vi "TSM SSC Digital Apply TDR Offsets Per-Site Per-Pin.vi"(0 "Digital TSM In":T1, 5 "Per-Site Per-Pin TDR Values":dbl[][](array[numeric]) format="%#_6p", 11 "error in":errorcluster) -> (4 "Digital TSM Out":T1, 15 "error out":errorcluster)   [LabVIEW 2020]
doc: "Applies the correction for propagation delay offsets to a digital pattern instrument. Use this VI to apply TDR offsets that are stored from a past measurement or are measured by means other than the niDigital TDR VI. Also use this VI to apply correction for offsets if the <B>apply offsets</B> input of the niDigital TDR VI was set to False at the time of measurement."
uses:
  TSM/TSM SSC Digital.ctl
  <vilib>/NI_TestStand_SemiconductorModule/NI_TestStand_Semiconductor_Module.lvlibp/PinMap/Digital Pattern/PinQueryContext/DigitalPatternPinQueryContext.lvclass
  SSC Digital/SSC Digital.ctl
  1a9f9ff5-721a-42b6-b454-8659b893b2e8.vi
  Shared SubVIs/Channel List to Pins.vi
  Shared SubVIs/Trim Whitespace [Inlined].vi
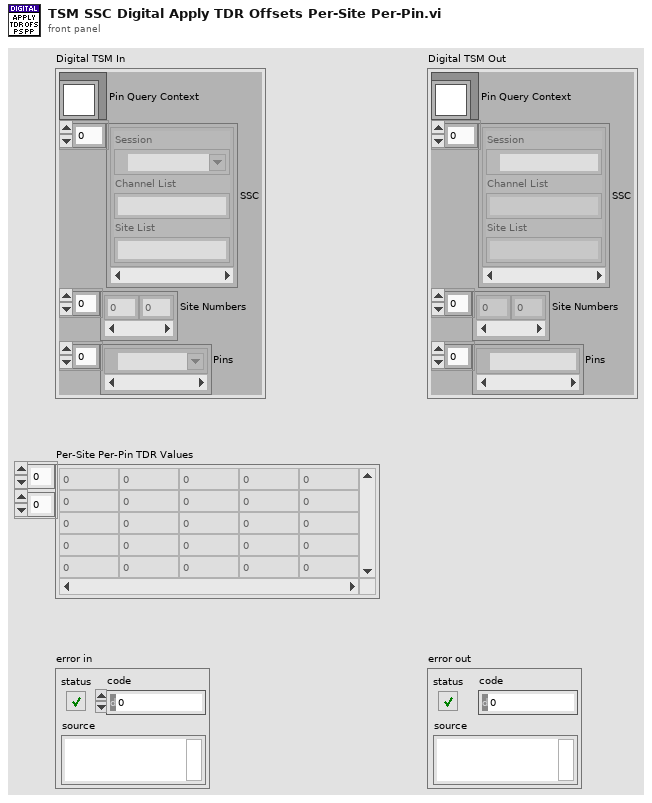
[diagram p1: front panel]
types:
  T1 = typedef "TSM SSC Digital.ctl" = cluster{"Pin Query Context":refnum<class "DigitalPatternPinQueryContext.lvclass">, "SSC":T2[], "Site Numbers":i32[], "Pins":tag[]}
  T2 = typedef "SSC Digital.ctl" = cluster{"Session":refnum<k15>, "Channel List":string, "Site List":string}
  T3 = typedef "Digital 2D Location.ctl" = cluster{"Row":i32, "Col":i32}
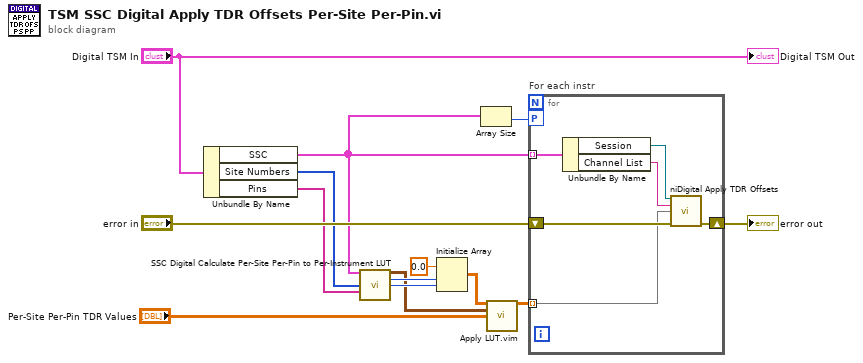
[diagram p0: block diagram]
diagram:
  n1 = Unbundle By Name("Digital TSM In") -> ("SSC"=w1:T2[], "Site Numbers"=w7:i32[], "Pins"=w6:tag[])
  n2 = call "SSC Digital Calculate Per-Site Per-Pin to Per-Instrument LUT.vi"("Digital SSC In"=w1, "Sites"=w7, "Pins"=w6) -> ("Per-Site Per-Pin to Per-Instrument LUT"=w10:T3[][], "Instrument Count"=w13:i32, "Max Sites on Instrument"=w12:i32)  [unwired: 10 in]
  n3 = Initialize Array(0.0 ("element"), w13, w12) -> (w11:dbl[][])
  n4 = Array Size(array=w1) -> (size(s)=w2:i32)
  n5 = call "Apply LUT.vim"("Initialized Array"=w11, "LUT"=w10, "Results to Apply LUT to"="Per-Site Per-Pin TDR Values") -> ("Array Out"=w9:dbl[][])  [unwired: 12 in]
  n6 = for "For each instr" {
    workers-P: w2 -> [_]
    tunnel: w1 -> [w17] mode=indexing
    tunnel: w9 -> [w18] mode=indexing
    shift-right: [w19] -> w3
    shift-left: "error in" -> [w20]
    n7 = Unbundle By Name(w17) -> ("Session"=w16:refnum<k15>, "Channel List"=w15:string)
    n8 = call <instrlib>:"niDigital Apply TDR Offsets.vi"("instrument handle"=w16, "channel list"=w15, "offsets (s)"=w18, "error in"=w20) -> ("error out"=w19:errorcluster)  [unwired: 10 in, 1 out]
  }
  "error out" <- w3
  "Digital TSM Out" <- "Digital TSM In"
